vi "LS1.vi"(5 "LS2":bool, 7 "LS3":bool, 9 "LS4":bool, 11 "LS5":bool) -> (6 "State Selector":T1)   [LabVIEW 2017]
uses:
  state_R.ctl
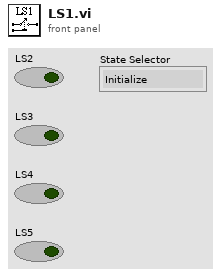
[diagram p1: front panel]
types:
  T1 = typedef "state_R.ctl" = enum16{"Initialize", "State 1", "State 2", "State 3", "State 4", "State 5", "State 6", "State 7", "State 8", "State 9", "UP", "DOWN", "EXTEND", "BACK", "Reset", "Process", "PAUSE", "Report", "Halt", "Shutdown"}
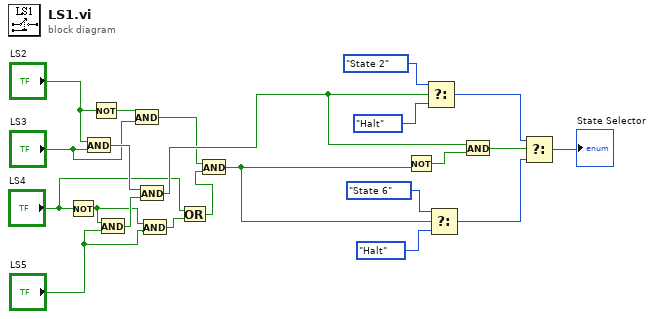
[diagram p0: block diagram]
diagram:
  n1 = Not(x="LS4") -> (.not. x?=w7:bool)
  n2 = And(x="LS2", y="LS3") -> (x .and. y?=w11:bool)
  n3 = Not(x="LS2") -> (.not. x?=w4:bool)
  n4 = And(x=w7, y="LS5") -> (x .and. y?=w12:bool)
  n5 = And(x=w4, y="LS3") -> (x .and. y?=w19:bool)
  n6 = And(x=w11, y=w12) -> (x .and. y?=w20:bool)
  n7 = And(x=w7, y="LS5") -> (x .and. y?=w9:bool)
  n8 = Or(x="LS4", y=w9) -> (x .or. y?=w8:bool)
  n9 = And(x=w19, y=w8) -> (x .and. y?=w1:bool)
  n10 = Not(x=w1) -> (.not. x?=w3:bool)
  n11 = Select(t=state_R."State 2" ("State Selector"), s=w20, f=state_R."Halt" ("State Selector")) -> (s? t:f=w17:T1)
  n12 = Select(t=state_R."State 6" ("State Selector"), s=w1, f=state_R."Halt" ("State Selector")) -> (s? t:f=w18:T1)
  n13 = And(x=w20, y=w3) -> (x .and. y?=w21:bool)
  n14 = Select(t=w17, s=w21, f=w18) -> (s? t:f=→"State Selector":T1)
